vi "Normalize Maud's PSD Signals.vi"(1 "Raw PSD voltages\n(Vc diff, Va diff, Vc sum, Va sum)":dbl[][](array[numeric])) -> (0 "amplified and\nnormalized signals\n(Vc norm, Va norm,\nVc diff, Va diff,\nVc sum, Va sum)":dbl[][](array[numeric]))   [LabVIEW 2017]
panel:
  in  "Vc sum gain":dbl=-1.0
  in  "Vc sum trim":dbl=0.0012
  in  "Va sum trim":dbl=-0.086
  in  "Va sum gain":dbl=1.0
  in  "Va diff gain":dbl=30.0
  in  "Va diff trim":dbl=-1.29
  in  "Vc diff trim":dbl=-3.97
  in  "Vc diff gain":dbl=30.0
  # "INPUTS:"
  # "OUTPUTS:"
  # "NOTE:  Maud's\nsignals are assumed\nto correspond to\nthe last four arrays\n(i.e., 4 through 7,\ncontaining Vc diff,\nVa diff, Vc sum, and\nVa sum, respectively).\n\nThe first four arrays,\nwhich should carry\nOscar's signals, are\nignored in this subVI."
  # "MAUD's ADJUSTMENTS:"
  # "20_0914: Chip copied\nthese adjustments\nfrom Maud"
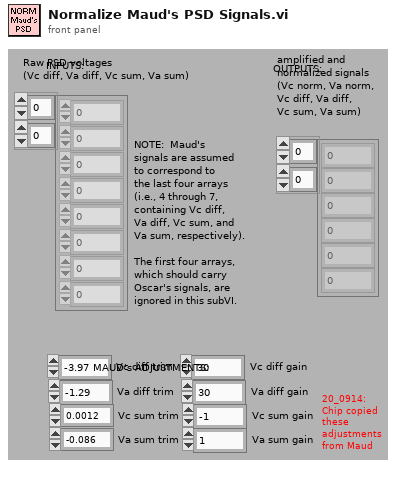
[diagram p1: front panel]
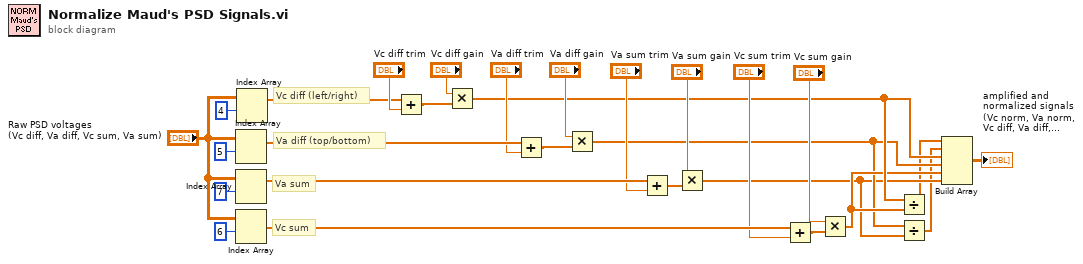
[diagram p0: block diagram]
diagram:
  # "Vc diff (left/right)"
  # "Va diff (top/bottom)"
  # "Va sum"
  # "Vc sum"
  n1 = Index Array(array="Raw PSD voltages\n(Vc diff, Va diff, Vc sum, Va sum)", index (row)=5 ("index")) -> (element=w18:dbl[])  [unwired: 1 in]
  n2 = Index Array(array="Raw PSD voltages\n(Vc diff, Va diff, Vc sum, Va sum)", index (row)=7 ("index")) -> (element=w14:dbl[])  [unwired: 1 in]
  n3 = Index Array(array="Raw PSD voltages\n(Vc diff, Va diff, Vc sum, Va sum)", index (row)=6 ("index")) -> (element=w12:dbl[])  [unwired: 1 in]
  n4 = Index Array(array="Raw PSD voltages\n(Vc diff, Va diff, Vc sum, Va sum)", index (row)=4 ("index")) -> (element=w21:dbl[])  [unwired: 1 in]
  n5 = Add(x=w21, y="Vc diff trim") -> (x+y=w20:dbl[])
  n6 = Multiply(x="Vc diff gain", y=w20) -> (x*y=w7:dbl[])
  n7 = Add(x=w18, y="Va diff trim") -> (x+y=w19:dbl[])
  n8 = Multiply(x="Va diff gain", y=w19) -> (x*y=w5:dbl[])
  n9 = Add(x=w14, y="Va sum trim") -> (x+y=w15:dbl[])
  n10 = Multiply(x="Va sum gain", y=w15) -> (x*y=w4:dbl[])
  n11 = Add(x=w12, y="Vc sum trim") -> (x+y=w13:dbl[])
  n12 = Multiply(x="Vc sum gain", y=w13) -> (x*y=w6:dbl[])
  n13 = Divide(x=w7, y=w6) -> (x/y=w2:dbl[])
  n14 = Divide(x=w5, y=w4) -> (x/y=w1:dbl[])
  n15 = Build Array(w2, w1, w7, w5, w6, w4) -> (→"amplified and\nnormalized signals\n(Vc norm, Va norm,\nVc diff, Va diff,\nVc sum, Va sum)":dbl[][])
